vi "K_S30_VISA Global.vi"() -> ()   [LabVIEW 2012]
panel:
  in  "RS-converter:\necho":bool=TRUE
  in  "VISA resource":refnum<visa-resource-name>="COM2"
  # "Global Variable for KELLER S30 driver Labview"
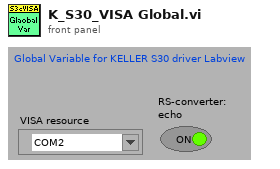
[diagram p1: front panel]
diagram:
